vi "Set Version in titlebar.vi"(5 "error in (no error)":errorcluster, 6 "Version":string, 8 "VI to set":refnum<vi>) -> (0 "error out":errorcluster, 3 "reference out":refnum<vi>)   [LabVIEW 2013]
doc: "This .vi appends the Version string to the title bar text in the specified .vi"
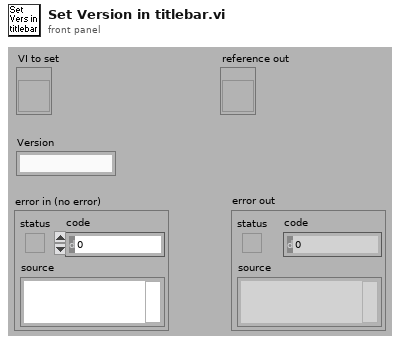
[diagram p1: front panel]
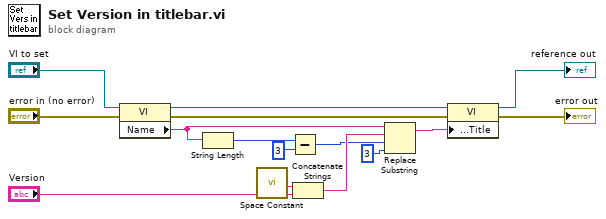
[diagram p0: block diagram]
diagram:
  n1 = property class="VI"(reference="VI to set", error in="error in (no error)") -> (reference out=w6:refnum<vi>, error out=w3:errorcluster, "Name"=w9:string)
  n2 = String Length(string=w9) -> (length=w7:i32)
  n3 = call <vilib>:"Space Constant.vi"() -> ("String"=w15:string)
  n4 = Subtract(x=w7, y=3) -> (x-y=w10:i32)
  n5 = Concatenate Strings(w15, "Version") -> (w14:string)
  n6 = Replace Substring(2:3 ("length (len. of substring)"), 3:w10, 4:w14, 5:w9) -> (1:w11:string)  [unwired: 1 out]
  n7 = property class="VI"(reference=w6, error in=w3, "Front Panel.Title"=w11) -> (reference out=→"reference out":refnum<vi>, error out=→"error out":errorcluster)
